vi "BotSpeak_Set.vi"(2 "value":string="0", 3 "Variable In":string="power", 4 "Bot Settings":T1) -> (1 "Bot Settings":T1)   [LabVIEW 2012]
doc: "Sets the value of \"Variable in\" and returns that as \"value\"."
uses:
  <userlib>/botspeak/VIs/Direct/BotSpeak_Control.ctl
panel:
  out "response":string
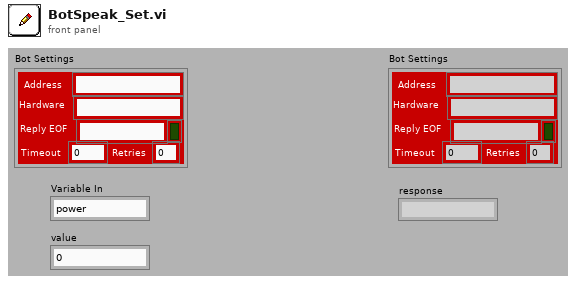
[diagram p1: front panel]
types:
  T1 = typedef "BotSpeak_Control.ctl" = cluster{"Address":string, "Reply EOF":string, "Hardware":string, "Retries":i8, "Timeout":i32, "Open?":bool}
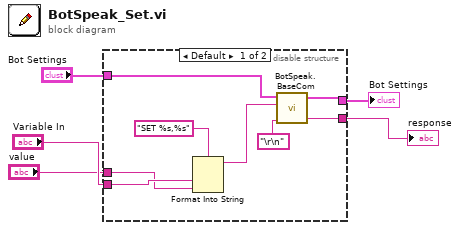
[diagram p0: block diagram]
diagram:
  n1 = disable-structure shown="Default" {
    disable-tunnel: "Bot Settings" -> [w11 _]
    disable-tunnel: [w10 _] -> w4
    disable-tunnel: "Variable In" -> [w9 _]
    disable-tunnel: "value" -> [w8 _]
    disable-tunnel: [w7 _] -> w1
    frame condition #0 (active) {
      n2 = Format Into String(format string="SET %s,%s" ("command"), w9, w8) -> (resulting string=w13:string)  [unwired: 2 in, 1 out]
      n3 = call <userlib>:"BotSpeak.BaseCom.vi"("Termination"="\r\n", "command"=w13, "Bot Settings in"=w11) -> ("response"=w7:string, "Bot Settings out"=w10:T1)  [unwired: 2 in]
    }
    frame condition #1 {
    }
  }
  "Bot Settings" <- w4
  "response" <- w1
